vi "Write Imaging Data.vi"(10 "Address":u32, 11 "packer out":T1) -> ()   [LabVIEW 2015]
uses:
  <vilib>/rvi/Memory/Memory_Emulation/niFpgaMemoryFastEmulationDramWriteAndRequestData.vi
  <vilib>/rvi/Memory/Memory_Emulation/niFpgaMemoryEmulationDramWriteAndRequestData.vi
  <vilib>/rvi/DataTransferAndStorage/Container/Common/niFpgaContainerGetUniqueNameForEmu.vi
  <vilib>/rvi/Memory/Memory_Emulation/niFpgaMemoryEmulationDramWriteAndRequestDataApplyByteEnables.vi
  <vilib>/rvi/DataTransferAndStorage/Container/XNode/niFpgaContainer.xnode
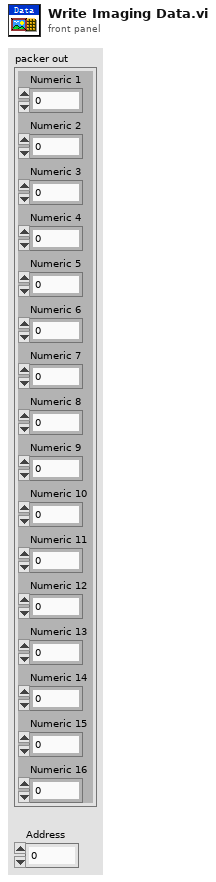
[diagram p1: front panel]
types:
  T1 = cluster{"Numeric 1":u32, "Numeric 2":u32, "Numeric 3":u32, "Numeric 4":u32, "Numeric 5":u32, "Numeric 6":u32, "Numeric 7":u32, "Numeric 8":u32, "Numeric 9":u32, "Numeric 10":u32, "Numeric 11":u32, "Numeric 12":u32, "Numeric 13":u32, "Numeric 14":u32, "Numeric 15":u32, "Numeric 16":u32}
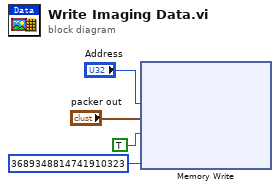
[diagram p0: block diagram]
diagram:
  n1 = xnode ("Memory Write")("Address"="Address", "Data"="packer out", "Input Valid"=TRUE, "Byte Enables"=i64 3689348814741910323) -> ()  [unwired: 1 in, 2 out]
